vi "plotStyle.vi"(11 "plotSpec":T1={"Style"="linespoints", "Color"=0, "PointType"=1, "PointSize"=1.0, "LineWidth"=1.0, "LineType"=1} {"LineType" min=1 max=6 step=1; "LineWidth" min=1 max=6 step=1; "PointSize" min=0 step=0.1}) -> (3 "String":string)   [LabVIEW 2014]
uses:
  plotstyle.ctl
panel:
  # "Style                      Colour    PointType       PointSize         Linewidth     Linestyle"
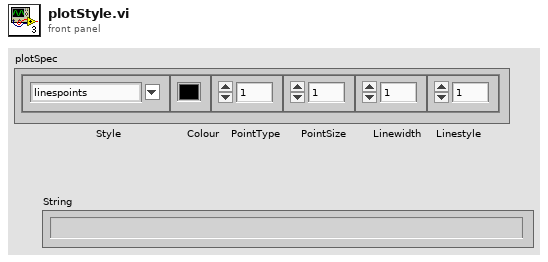
[diagram p1: front panel]
types:
  T1 = typedef "plotstyle.ctl" = cluster{"Style":string, "Color":u32, "PointType":i32, "PointSize":sgl, "LineWidth":sgl, "LineType":u8}
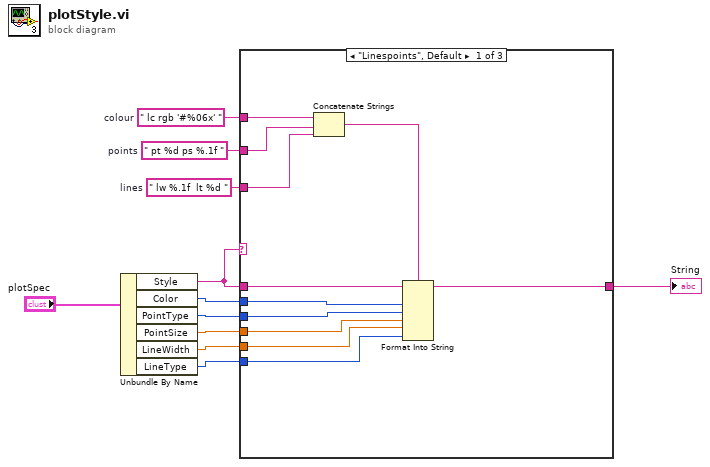
[diagram p0: block diagram]
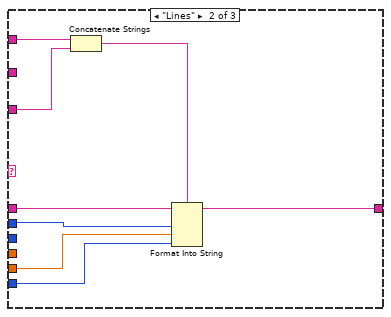
[diagram p2: hidden frame]
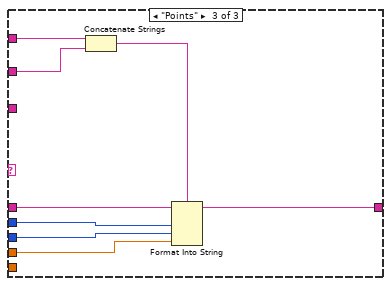
[diagram p3: hidden frame]
diagram:
  w5 = " lc rgb '#%06x' "  # colour
  w3 = " lw %.1f  lt %d "  # lines
  w4 = " pt %d ps %.1f "  # points
  n1 = Unbundle By Name("plotSpec") -> ("Style"=w10:string, "Color"=w11:u32, "PointType"=w8:i32, "PointSize"=w9:sgl, "LineWidth"=w1:sgl, "LineType"=w2:u8)
  n2 = case shown="\"Linespoints\", Default" w10 {
    tunnel: [w22 w30 w38] -> w7
    tunnel: w10 -> [w21 w29 w37]
    tunnel: w11 -> [w20 w28 w36]
    tunnel: w8 -> [w19 _ w35]
    tunnel: w9 -> [w18 _ w34]
    tunnel: w5 -> [w17 w27 w33]
    tunnel: w4 -> [w16 _ w32]
    tunnel: w3 -> [w15 w26 _]
    tunnel: w2 -> [w12 w24 _]
    tunnel: w1 -> [w13 w23 _]
    frame "Linespoints", Default {
      n3 = Concatenate Strings(w17, w16, w15) -> (w14:string)
      n4 = Format Into String(format string=w14, initial string=w21, w20, w19, w18, w13, w12) -> (resulting string=w22:string)  [unwired: 1 in, 1 out]
    }
    frame "Lines" {
      n5 = Concatenate Strings(w27, w26) -> (w25:string)
      n6 = Format Into String(format string=w25, initial string=w29, w28, w23, w24) -> (resulting string=w30:string)  [unwired: 1 in, 1 out]
    }
    frame "Points" {
      n7 = Concatenate Strings(w33, w32) -> (w31:string)
      n8 = Format Into String(format string=w31, initial string=w37, w36, w35, w34) -> (resulting string=w38:string)  [unwired: 1 in, 1 out]
    }
  }
  "String" <- w7
